vi "BuildHistoryCluster.vi"(7 "NewValueWeighting":dbl, 9 "NoiseFloorSum":dbl, 10 "Channel Power Beac":dbl, 11 "Channel Power Cal":dbl) -> (3 "output cluster":T1)   [LabVIEW 2018]
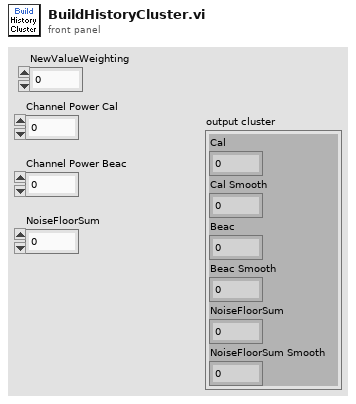
[diagram p1: front panel]
types:
  T1 = cluster{"Cal":dbl, "Cal Smooth":dbl, "Beac":dbl, "Beac Smooth":dbl, "NoiseFloorSum":dbl, "NoiseFloorSum Smooth":dbl}
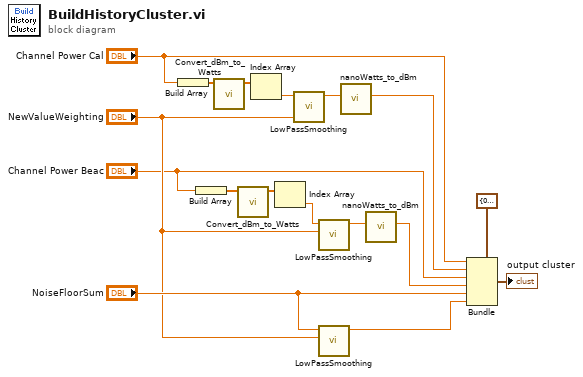
[diagram p0: block diagram]
diagram:
  n1 = Build Array("Channel Power Cal") -> (w11:dbl[])
  n2 = Build Array("Channel Power Beac") -> (w8:dbl[])
  n3 = call "Convert_dBm_to_Watts.vi"("P(dBm)"=w11) -> ("P(n_watts)"=w12:dbl[])  [unwired: 10 in]
  n4 = call "Convert_dBm_to_Watts.vi"("P(dBm)"=w8) -> ("P(n_watts)"=w7:dbl[])  [unwired: 10 in]
  n5 = Index Array(array=w12) -> (element=w9:dbl)  [unwired: 1 in]
  n6 = Index Array(array=w7) -> (element=w5:dbl)  [unwired: 1 in]
  n7 = call "LowPassSmoothing.vi"("NewValueWeighting"="NewValueWeighting", "New Value"=w9) -> ("Filtered Value"=w4:dbl)  [unwired: 9 in]
  n8 = call "LowPassSmoothing.vi"("NewValueWeighting"="NewValueWeighting", "New Value"=w5) -> ("Filtered Value"=w2:dbl)  [unwired: 9 in]
  n9 = call "LowPassSmoothing.vi"("NewValueWeighting"="NewValueWeighting", "New Value"="NoiseFloorSum") -> ("Filtered Value"=w14:dbl)  [unwired: 9 in]
  n10 = call "nanoWatts_to_dBm.vi"("P(nW)"=w4) -> ("dBm"=w3:dbl)  [unwired: 10 in]
  n11 = call "nanoWatts_to_dBm.vi"("P(nW)"=w2) -> ("dBm"=w1:dbl)  [unwired: 10 in]
  n12 = Bundle(cluster=T1 {"Cal"=0.0, "Cal Smooth"=0.0, "Beac"=0.0, "Beac Smooth"=0.0, "NoiseFloorSum"=0.0, "NoiseFloorSum Smooth"=0.0}, "Cal"="Channel Power Cal", "Cal Smooth"=w3, "Beac"="Channel Power Beac", "Beac Smooth"=w1, "NoiseFloorSum"="NoiseFloorSum", "NoiseFloorSum Smooth"=w14) -> (→"output cluster":T1)
